vi "ArmResetI.vi"(9 "Disabled?":bool, 11 "ArmState":T1=enum."1 Tote") -> (7 "Reset I":bool)   [LabVIEW 2014]
uses:
  Typedefs/Arm States.ctl
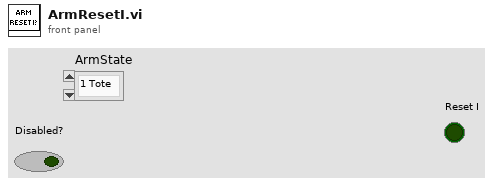
[diagram p1: front panel]
types:
  T1 = typedef "Arm States.ctl" = enum16{"Arm Manual ", "Ground", "Step", "1 Tote", "2 Tote", "3 Tote", "4 Tote", "5 Tote", "6 Tote", "Flip Can Arm", "Grab Can in auto", "Nudge"}
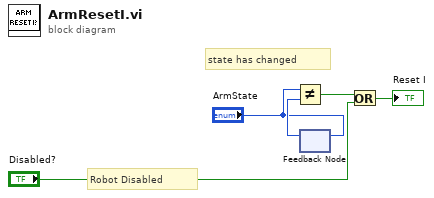
[diagram p0: block diagram]
diagram:
  # "Robot Disabled"
  # "state has changed"
  n1 = feedback #1() -> (w2:T1)  [unwired: 1 in]
  n2 = Not Equal?(x="ArmState", y=w2) -> (x != y?=w4:bool)
  n3 = feedback-in #1("ArmState") -> ()
  n4 = Or(x=w4, y="Disabled?") -> (x .or. y?=→"Reset I":bool)
